vi "Generate Clock using Metronome - cRIO.vi"() -> ()   [LabVIEW 2020]
uses:
  FPGA Timekeeper.lvlib
  <vilib>/eio/EIONode/EIONode.xnode
panel:
  in  "clock high duration (ns)":u32=500000000
  in  "clock period (ns)":u32=1000000000
  in  "clock start time (ns)":u64
  in  "enable clock generation":bool
  out "offset from time reference":i32
  out "FPGA Timekeeper locked":bool
  out "FPGA Timekeeper time (ns)":u64
  # "This example generates a clock using the Metronome VI of the FPGA Timekeeper API."
  # "The default values for the controls clock high duration (ns), clock period (ns), and clock start time (ns) will generate a clock frequency of 1 Hz with a 50% duty cycle with the rising edge aligned to the beginning of each second."
  # "Clock Generation"
  # "FPGA Timekeeper"
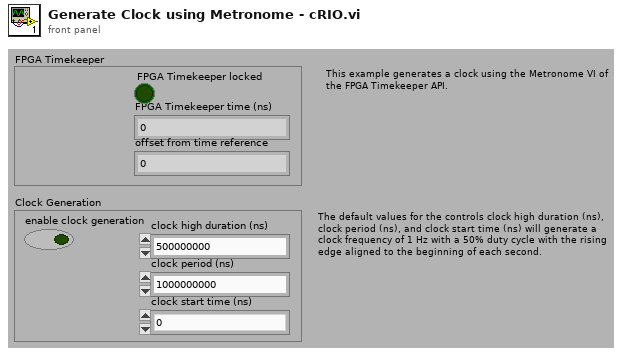
[diagram p1: front panel]
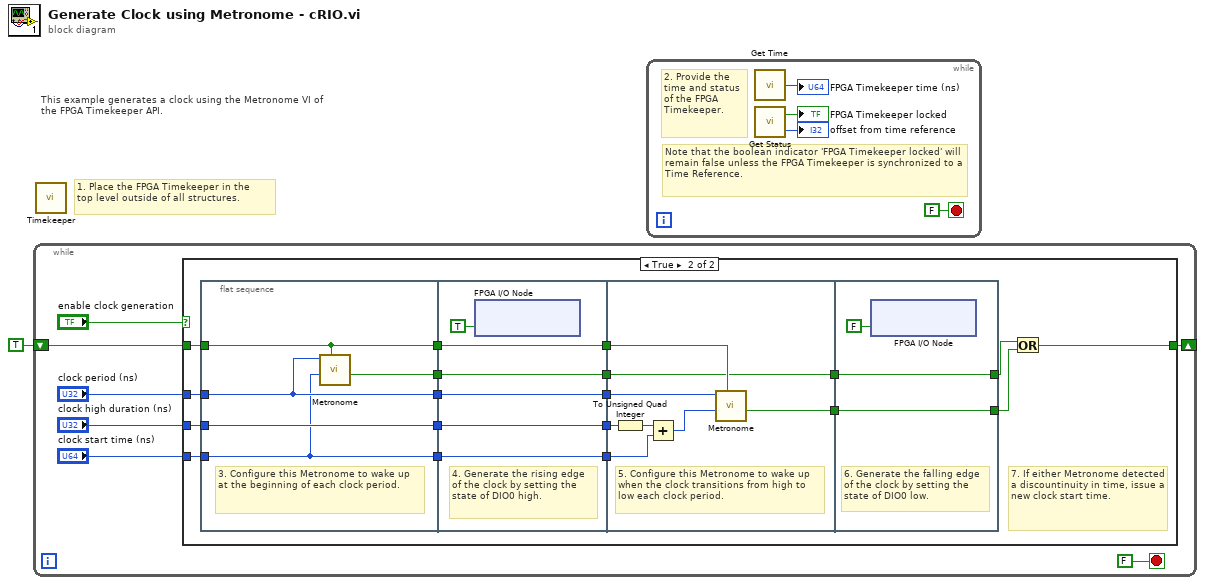
[diagram p0: block diagram]
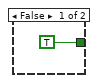
[diagram p2: hidden frame]
diagram:
  # "This example generates a clock using the Metronome VI of the FPGA Timekeeper API."
  # "1. Place the FPGA Timekeeper in the\ntop level outside of all structures."
  n1 = while {
    shift-right: [w6] -> _
    shift-left: TRUE ("Time Snapped Event") -> [w7]
    stop <- FALSE stop-if-true
    n2 = case shown="True" "enable clock generation" {
      tunnel: w7 -> [_ w28]
      tunnel: [TRUE w10] -> w6
      tunnel: "clock period (ns)" -> [_ w19]
      tunnel: "clock high duration (ns)" -> [_ w24]
      tunnel: "clock start time (ns)" -> [_ w25]
      frame False {
      }
      frame True {
        # "7. If either Metronome detected a discountinuity in time, issue a new clock start time."
        n3 = flat-sequence {
          tunnel: w28 -> [w33]
          tunnel: [w33] -> w26
          tunnel: w25 -> [w30]
          tunnel: w24 -> [w32]
          tunnel: [w32] -> w23
          tunnel: [w30] -> w21
          tunnel: w19 -> [w31]
          tunnel: [w31] -> w18
          tunnel: [w29] -> w16
          tunnel: [w39] -> w27
          tunnel: w26 -> [w39]
          tunnel: w23 -> [w38]
          tunnel: [w38] -> w22
          tunnel: w21 -> [w37]
          tunnel: [w37] -> w20
          tunnel: w18 -> [w35]
          tunnel: [w35] -> w17
          tunnel: w16 -> [w34]
          tunnel: [w34] -> w15
          tunnel: w27 -> [w47]
          tunnel: w22 -> [w44]
          tunnel: w20 -> [w43]
          tunnel: w17 -> [w42]
          tunnel: w15 -> [w41]
          tunnel: [w41] -> w14
          tunnel: [w40] -> w13
          tunnel: w14 -> [w49]
          tunnel: w13 -> [w48]
          tunnel: [w49] -> w12
          tunnel: [w48] -> w11
          frame #0 {
            # "3. Configure this Metronome to wake up at the beginning of each clock period."
            n4 = call "Metronome.vi"("initialize"=w33, "start time (ns)"=w30, "loop period (ns)"=w31) -> ("time snapped event"=w29:bool)  [unwired: 5 in, 1 out]
          }
          frame #1 {
            # "4. Generate the rising edge of the clock by setting the state of DIO0 high."
            n5 = xnode "FPGA I/O Node"("Mod1/DIO0"=TRUE) -> ()  [unwired: 1 in, 1 out]
          }
          frame #2 {
            # "5. Configure this Metronome to wake up when the clock transitions from high to low each clock period."
            n6 = To Unsigned Quad Integer(1:w44) -> (0:w46:u64)
            n7 = Add(x=w46, y=w43) -> (x+y=w45:u64)
            n8 = call "Metronome.vi"("initialize"=w47, "start time (ns)"=w45, "loop period (ns)"=w42) -> ("time snapped event"=w40:bool)  [unwired: 5 in, 1 out]
          }
          frame #3 {
            # "6. Generate the falling edge of the clock by setting the state of DIO0 low."
            n9 = xnode "FPGA I/O Node"("Mod1/DIO0"=FALSE) -> ()  [unwired: 1 in, 1 out]
          }
        }
        n10 = Or(x=w12, y=w11) -> (x .or. y?=w10:bool)
      }
    }
  }
  n11 = call "Timekeeper.vi"() -> ()  [unwired: 12 in]
  n12 = while {
    stop <- FALSE stop-if-true
    # "Note that the boolean indicator 'FPGA Timekeeper locked' will \nremain false unless the FPGA Timekeeper is synchronized to a Time Reference."
    # "2. Provide the time and status of the FPGA Timekeeper."
    n13 = call "Get Time.vi"() -> ("time (ns)"=→"FPGA Timekeeper time (ns)":u64)
    n14 = call "Get Status.vi"() -> ("FPGA Timekeeper locked"=→"FPGA Timekeeper locked":bool, "offset from time reference"=→"offset from time reference":i32)
  }
